vi "GetCollisions.vi"(8 "error in (no error)":errorcluster, 11 "Level in":refnum<class "Level.lvclass">) -> (0 "error out":errorcluster, 2 "Collisions":T1[](array[typedef]), 3 "Level out":refnum<class "Level.lvclass">)   [LabVIEW 2015, in "Level.lvclass"]
uses:
  Level.lvclass
  Segment.ctl
  Point.ctl
  Level.lvclass/Level.ctl
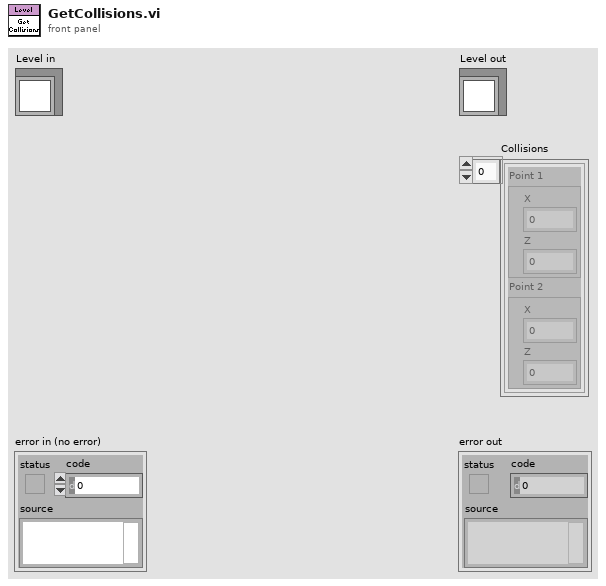
[diagram p1: front panel]
types:
  T1 = typedef "Level.lvclass/Segment.ctl" = cluster{"Point 1":T2, "Point 2":T2}
  T2 = typedef "Level.lvclass/Point.ctl" = cluster{"Z":dbl, "X":dbl}
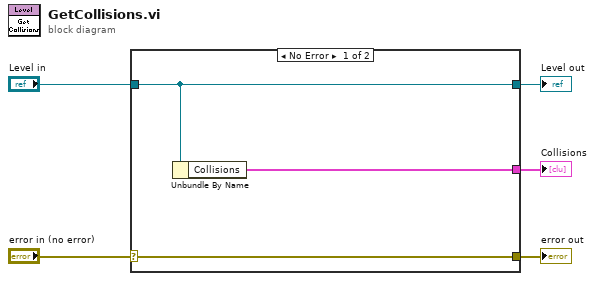
[diagram p0: block diagram]
diagram:
  n1 = case shown="No Error" "error in (no error)" {
    selector: "error in (no error)" -> [w8 w9]
    tunnel: [w8 w9] -> w4
    tunnel: [w7 w10] -> w2
    tunnel: "Level in" -> [w7 w10]
    tunnel: [w6 _] -> w1
    frame No Error {
      n2 = Unbundle By Name(w7) -> ("Collisions"=w6:T1[])
    }
    frame Error {
    }
  }
  "error out" <- w4
  "Level out" <- w2
  "Collisions" <- w1
